vi "Write Socket.vi"(8 "error in (no error)":errorcluster, 10 "Socket":refnum<class "Socket.lvclass">, 11 "WebSocket in":refnum<class "WebSocket.lvclass">) -> (0 "error out":errorcluster, 3 "WebSocket out":refnum<class "WebSocket.lvclass">)   [LabVIEW 2021, in "WebSockets.lvlib" / "WebSocket.lvclass"]
doc: "Write the underlying socket object to the WebSocket connection.\nWebSockets 2.0.1.40\nSam Sharp - MediaMongrels Ltd\nCopyright (c) 2019, MediaMongrels Ltd"
uses:
  WebSocket.lvclass
  Sockets/Socket/Socket.lvclass
  WebSocket.lvclass/WebSocket.ctl
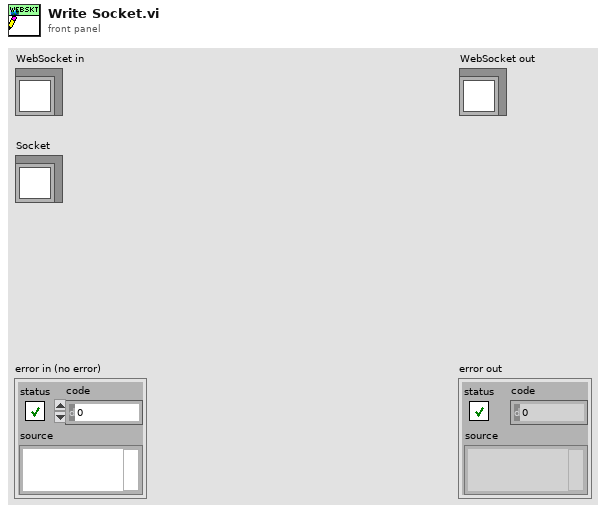
[diagram p1: front panel]
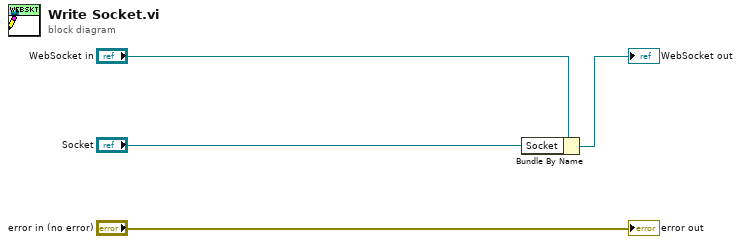
[diagram p0: block diagram]
diagram:
  n1 = Bundle By Name(cluster="WebSocket in", "Socket"="Socket") -> (→"WebSocket out":refnum<class "WebSocket.lvclass">)
  "error out" <- "error in (no error)"
